vi "Keys.vi"(8 "error in (no error)":errorcluster, 11 "StringMap in":refnum<class "StringMap.lvclass">) -> (0 "error out":errorcluster, 2 "Keys":string[](array[string]), 3 "StringMap out":refnum<class "StringMap.lvclass">)   [LabVIEW 2013, in "LapDog.Collections.v_.Maps.lvlib" / "StringMap.lvclass"]
doc: "Returns a copy of all keys in the map."
uses:
  StringMap.lvclass
  ObjectMap/ObjectMap.lvclass
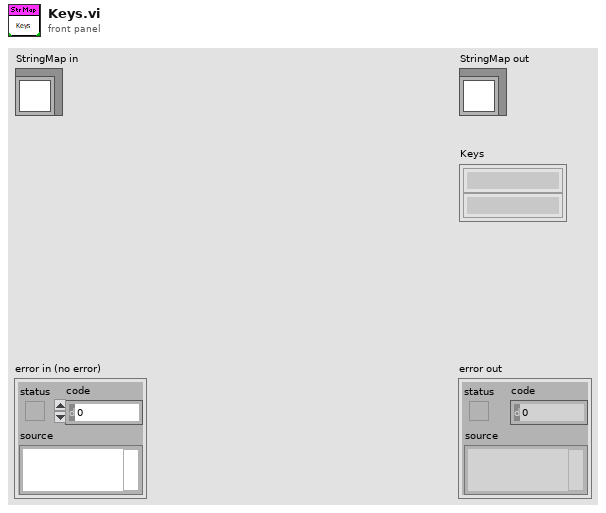
[diagram p1: front panel]
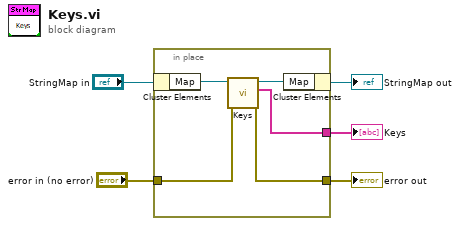
[diagram p0: block diagram]
diagram:
  n1 = in-place {
    in-place-border: "error in (no error)" -> [w8]
    in-place-border: [w7] -> w3
    in-place-border: [w6] -> w2
    n2 = in-place-cluster #1("StringMap in") -> ("Map"=w10:refnum<class "ObjectMap.lvclass">)
    n3 = call-dynamic "Keys.vi"("error in (no error)"=w8, "Map in"=w10) -> ("error out"=w7:errorcluster, "Keys"=w6:string[], "Map out"=w9:refnum<class "ObjectMap.lvclass">)  [unwired: 7 in]
    n4 = in-place-cluster #1("Map"=w9) -> (→"StringMap out":refnum<class "StringMap.lvclass">)
  }
  "error out" <- w3
  "Keys" <- w2
